vi "FCI 102 Lip Gap.vi"(0 "Image":T1, 5 "Lip Outer Points":cluster{"X":sgl, "Y":sgl}[](array[cluster]) {"Y" format="%.2f"; "X" format="%.2f"}, 7 "M ROI":T2, 9 "Calibrated Image":T1, 11 "error in (no error)":errorcluster) -> (4 "Image Out":T1, 6 "102 Lip Gap":sgl, 15 "error out":errorcluster)   [LabVIEW 2019, in "Algorithm.lvclass"]
uses:
  FrameworkOverrides/Algorithm.lvclass
  <vilib>/vision/NI_Vision_Development_Module.lvlib
  <vilib>/vision/Measure.llb/Edge Polarity.ctl
  <vilib>/vision/Measure.llb/Edge Options.ctl
  <vilib>/vision/Image Controls.llb/IMAQ Image.ctl
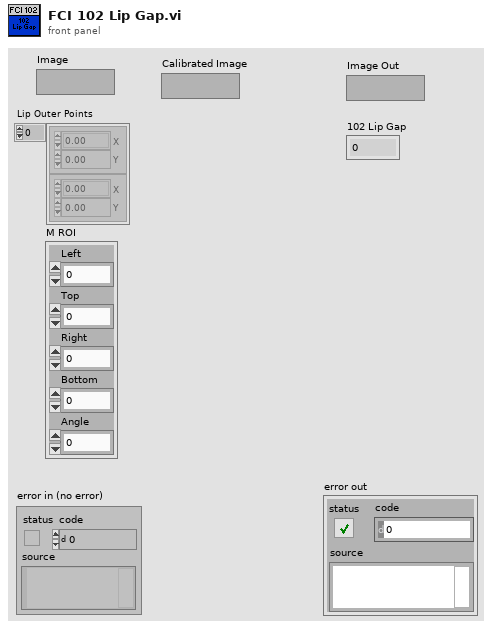
[diagram p1: front panel]
types:
  T1 = typedef "IMAQ Image.ctl" = refnum<image>
  T2 = cluster{"Left":dbl, "Top":dbl, "Right":dbl, "Bottom":dbl, "Angle":dbl}
  T3 = typedef "Edge Options.ctl" = cluster{"Edge Polarity":T4, "Kernel Size":u32, "Width":u32, "Minimum Edge Strength":sgl, "Interpolation Type":enum32{"Zero Order", "Bilinear", "Quadratic", "Cubic", "Bilinear Fixed"}, "Data Processing Method":enum32{"Average", "Median"}}
  T4 = typedef "Edge Polarity.ctl" = u32
  T5 = enum16{"Get First Edge", "Get First + Last Edge", "Get All Edges", "Get Best Edge"}
  T6 = typedef "ROI Descriptor" = cluster{"Global Rectangle":i32[], "Contours":cluster{"ID":enum32{"External", "Internal"}, "Type":u32, "Coordinates":i32[]}[]}
  T7 = typedef "Search Line.ctl" = cluster{"Start Point":cluster{"X":sgl, "Y":sgl}, "End Point":cluster{"X":sgl, "Y":sgl}, "Edge Info":T8[], "Edge Map":dbl[], "Calibration Valid":bool}
  T8 = typedef "Edge New.ctl" = cluster{"Location (Pixel)":cluster{"X":sgl, "Y":sgl}, "Location (Real-World)":cluster{"X":sgl, "Y":sgl}, "Distance (Pixel)":dbl, "Distance (Real-World)":dbl, "Strength":dbl, "Noise":dbl, "Rising?":bool}
  T9 = cluster{"First Edge Point":cluster{"X":sgl, "Y":sgl}, "Search Line First Edge":cluster{"X":sgl, "Y":sgl}}
  T10 = cluster{"Last Edge Point":cluster{"X":sgl, "Y":sgl}, "Search Line Last Edge":cluster{"X":sgl, "Y":sgl}}
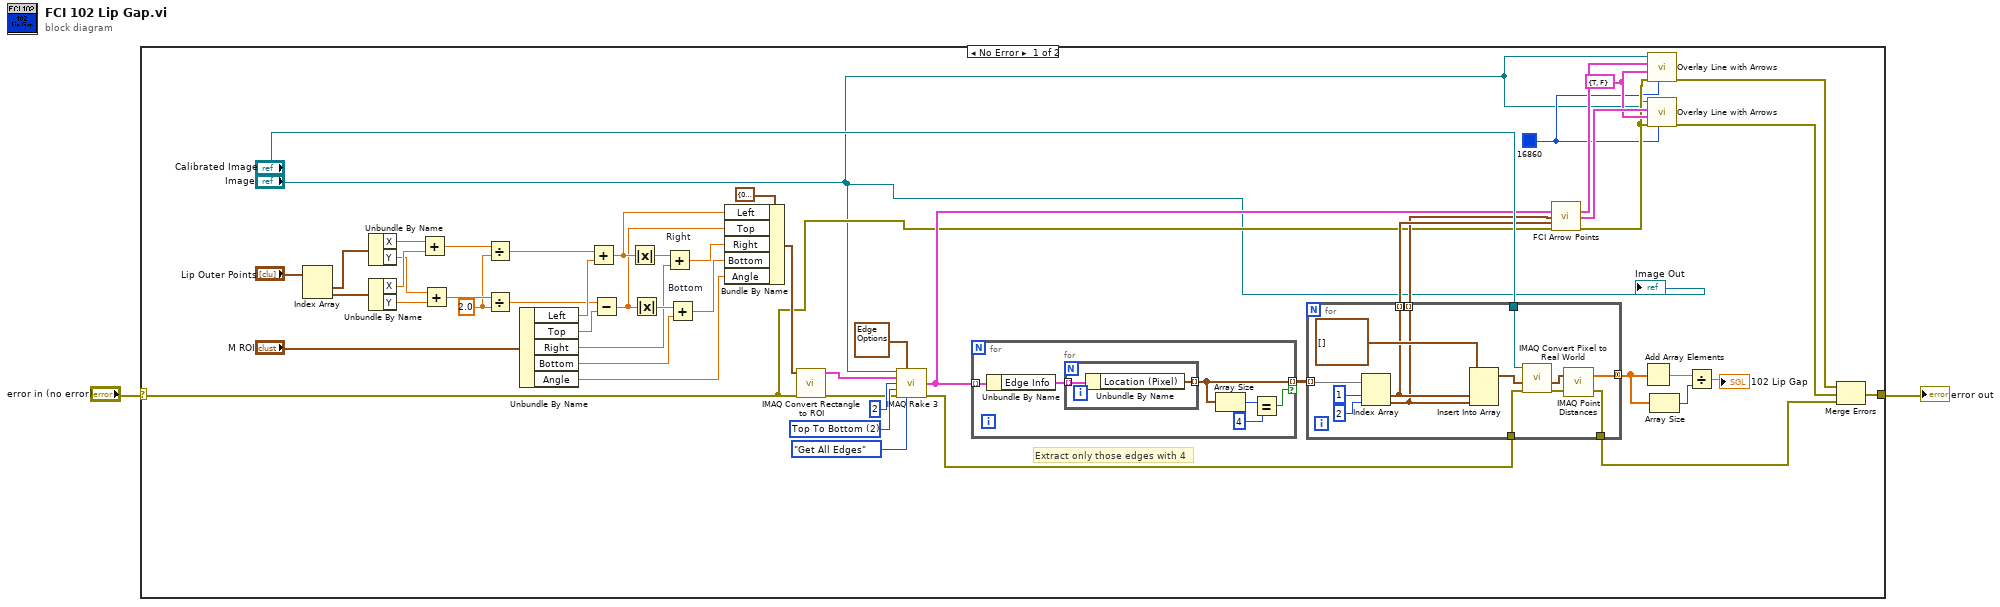
[diagram p0: block diagram]
diagram:
  n1 = case shown="No Error" "error in (no error)" {
    selector: "error in (no error)" -> [w4 w77]
    tunnel: [w7 w77] -> w1
    frame No Error {
      w12 = u32 16860 ("Color")
      w14 = cluster{"Start point":bool, "End point":bool} {"Start point"=TRUE, "End point"=FALSE} ("Arrows")
      w26 = u16 2 items=["Left To Right", "Right To Left", "Top To Bottom", "Bottom To Top"] ("Scan Direction")
      w49 = sgl 2.0 ("y")
      # "Extract only those edges with 4"
      n2 = Index Array(array="Lip Outer Points") -> (element #1=w47:cluster{"X":sgl, "Y":sgl}, element #2=w46:cluster{"X":sgl, "Y":sgl})  [unwired: 2 in]
      n3 = Unbundle By Name(w47) -> ("X"=w55:sgl, "Y"=w53:sgl)
      n4 = Unbundle By Name(w46) -> ("X"=w54:sgl, "Y"=w52:sgl)
      n5 = Add(x=w55, y=w54) -> (x+y=w51:sgl)
      n6 = Add(x=w53, y=w52) -> (x+y=w50:sgl)
      n7 = Divide(x=w51, y=w49) -> (x/y=w32:sgl)
      n8 = Divide(x=w50, y=w49) -> (x/y=w31:sgl)
      n9 = Unbundle By Name("M ROI") -> ("Left"=w38:dbl, "Top"=w37:dbl, "Right"=w36:dbl, "Bottom"=w35:dbl, "Angle"=w34:dbl)
      n10 = Add(x=w32, y=w38) -> (x+y=w42:dbl)
      n11 = Subtract(x=w31, y=w37) -> (x-y=w41:dbl)
      n12 = Absolute Value(x=w42) -> (abs(x)=w45:dbl)
      n13 = Absolute Value(x=w41) -> (abs(x)=w44:dbl)
      n14 = Add "Right"(x=w45, y=w36) -> (x+y=w40:dbl)
      n15 = Add "Bottom"(x=w44, y=w35) -> (x+y=w39:dbl)
      n16 = Bundle By Name(cluster=T2 {"Left"=0.0, "Top"=0.0, "Right"=0.0, "Bottom"=0.0, "Angle"=0.0} ("input cluster"), "Left"=w42, "Top"=w41, "Right"=w40, "Bottom"=w39, "Angle"=w34) -> (w33:T2)
      n17 = call "IMAQ Convert Rectangle to ROI"("error in (no error)"=w4, "Rectangle"=w33) -> ("error out"=w25:errorcluster, "ROI Descriptor"=w24:T6)  [unwired: 7 in]
      n18 = call "IMAQ Rake 3"("Image"="Image", "Edge Options"=T3 {"Edge Polarity"=0, "Kernel Size"=3, "Width"=3, "Minimum Edge Strength"=50.0, "Interpolation Type"=enum."Zero Order", "Data Processing Method"=enum."Average"}, "ROI Descriptor"=w24, "Step Size"=u32 2, "Scan Direction"=w26, "error in (no error)"=w25, "Process"=T5."Get All Edges") -> ("Search Lines"=w11:T7[], "error out"=w18:errorcluster)  [unwired: 5 in, 2 out]
      n19 = for {
        tunnel: w11 -> [w74] mode=indexing
        tunnel: [w72] -> w23 mode=indexing if=w70
        n20 = Unbundle By Name(w74) -> ("Edge Info"=w73:T8[])
        n21 = for {
          tunnel: w73 -> [w75] mode=indexing
          tunnel: [w76] -> w72 mode=indexing
          n22 = Unbundle By Name(w75) -> ("Location (Pixel)"=w76:cluster{"X":sgl, "Y":sgl})
        }
        n23 = Array Size(array=w72) -> (size(s)=w71:i32)
        n24 = Equal?(x=w71, y=4) -> (x = y?=w70:bool)
      }
      n25 = for {
        tunnel: w23 -> [w68] mode=indexing
        tunnel: [w64] -> w20 mode=concatenating
        tunnel: w18 -> [w59]
        tunnel: [w63] -> w8
        tunnel: "Calibrated Image" -> [w62]
        tunnel: [w57] -> w6 mode=indexing
        tunnel: [w56] -> w5 mode=indexing
        n26 = Index Array(array=w68, index #1=1 ("index"), index #2=2 ("index")) -> (element #1=w57:cluster{"X":sgl, "Y":sgl}, element #2=w56:cluster{"X":sgl, "Y":sgl})
        n27 = Insert Into Array(array=cluster{"X":sgl, "Y":sgl}[] [], new element #1=w57, new element #2=w56) -> (w61:cluster{"X":sgl, "Y":sgl}[])  [unwired: 1 in]
        n28 = call "IMAQ Convert Pixel to Real World"("error in (no error)"=w59, "Array of Pixel Coordinates"=w61, "Calibrated Image"=w62) -> ("error out"=w58:errorcluster, "Array of Real World Coordinates"=w60:cluster{"X":sgl, "Y":sgl}[])  [unwired: 3 in, 4 out]
        n29 = call "IMAQ Point Distances"("Points"=w60, "error in (no error)"=w58) -> ("Distances"=w64:sgl[], "error out"=w63:errorcluster)  [unwired: 3 in]
      }
      n30 = call "FCI Arrow Points.vi"("Search Lines"=w11, "Edge Last Points"=w5, "Edge First Points"=w6, "error constant"=w4) -> ("First Arrow Line Coord"=w16:T9, "Second Arrow Line Coord"=w15:T10, "error IO"=w13:errorcluster)  [unwired: 7 in, 2 out]
      n31 = Add Array Elements(numeric array=w20) -> (sum=w22:sgl)
      n32 = call <vilib>:"Overlay Line with Arrows.vi"("Color"=w12, "error in (no error)"=w13, "Arrows"=w14, "Line Coordinates"=w16, "Image In"="Image") -> ("error out"=w10:errorcluster)  [unwired: 5 in, 1 out]
      n33 = call <vilib>:"Overlay Line with Arrows.vi"("Color"=w12, "error in (no error)"=w13, "Arrows"=w14, "Line Coordinates"=w15, "Image In"="Image") -> ("error out"=w9:errorcluster)  [unwired: 5 in, 1 out]
      n34 = Array Size(array=w20) -> (size(s)=w19:i32)
      n35 = Divide(x=w22, y=w19) -> (x/y=→"102 Lip Gap":sgl)
      n36 = Merge Errors(w10, w9, w8) -> (w7:errorcluster)
      "Image Out" <- "Image"
    }
    frame Error {
    }
  }
  "error out" <- w1
